vi "Send Message.vi"(6 "timeout in ms (-1)":i32=-1, 8 "error in (no error)":errorcluster, 9 "Message in":refnum<class "Abstract Message.lvclass">, 10 "Consumer in":string, 11 "Abstract Producer in":refnum<class "Abstract Producer.lvclass">) -> (0 "error out":errorcluster, 1 "Message out":refnum<class "Abstract Message.lvclass">, 3 "Abstract Producer out":refnum<class "Abstract Producer.lvclass">, 4 "timed out?":bool)   [LabVIEW 2017, in "Messaging.lvlib" / "Abstract Producer.lvclass"]
uses:
  Abstract Producer.lvclass
  Message/Abstract Message/Abstract Message.lvclass
  Abstract Producer.lvclass/Abstract Producer.ctl
  Message Queue/Abstract Message Queue/Abstract Message Queue.lvclass
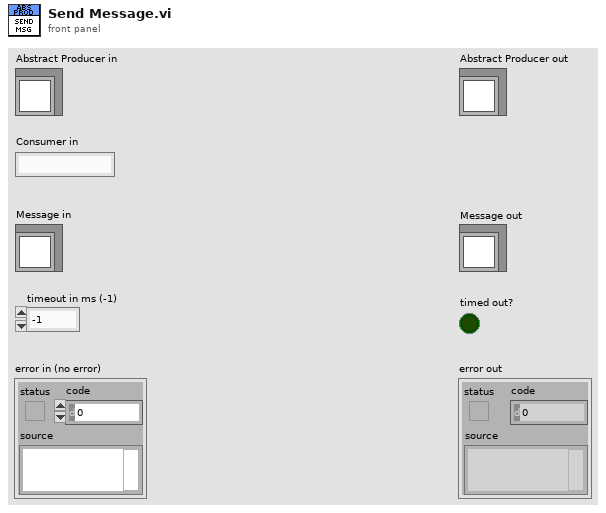
[diagram p1: front panel]
types:
  T1 = typedef "Messaging.lvlib/Abstract Producer.lvclass/Consumer Information.ctl" = cluster{"Name":string, "Request Queue":refnum<class "Abstract Message Queue.lvclass">, "Response Queue":refnum<class "Abstract Message Queue.lvclass">}
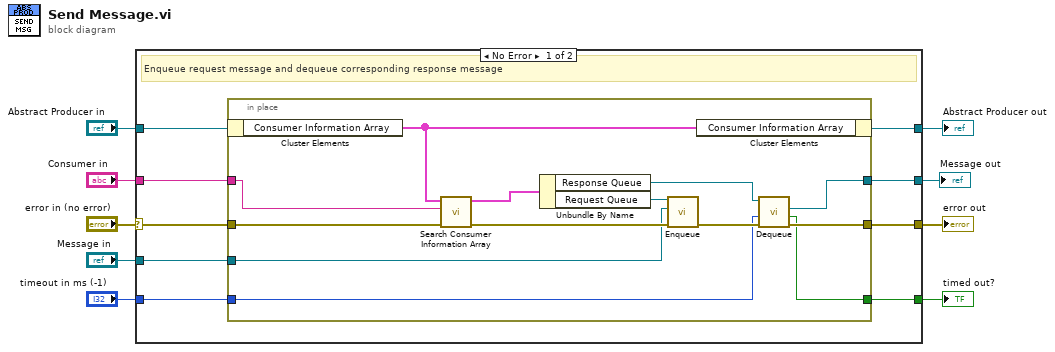
[diagram p0: block diagram]
diagram:
  n1 = case shown="No Error" "error in (no error)" {
    selector: "error in (no error)" -> [w14 w33]
    tunnel: [w13 w33] -> w8
    tunnel: [w17 w32] -> w6
    tunnel: "Abstract Producer in" -> [w18 w32]
    tunnel: "Consumer in" -> [w16 _]
    tunnel: "Message in" -> [w15 _]
    tunnel: [w12 _] -> w3
    tunnel: "timeout in ms (-1)" -> [w11 _]
    tunnel: [w10 _] -> w1
    frame No Error {
      # "Enqueue request message and dequeue corresponding response message"
      n2 = in-place {
        in-place-border: w16 -> [w31]
        in-place-border: w15 -> [w25]
        in-place-border: w14 -> [w29]
        in-place-border: [w23] -> w13
        in-place-border: [w21] -> w12
        in-place-border: w11 -> [w20]
        in-place-border: [w19] -> w10
        n3 = in-place-cluster #1(w18) -> ("Consumer Information Array"=w30:T1[])
        n4 = call "Search Consumer Information Array.vi"("error in (no error)"=w29, "Consumer in"=w31, "Consumer Information Array in"=w30) -> ("error out"=w28:errorcluster, "Consumer Information out"=w27:T1)  [unwired: 7 in]
        n5 = Unbundle By Name(w27) -> ("Response Queue"=w22:refnum<class "Abstract Message Queue.lvclass">, "Request Queue"=w26:refnum<class "Abstract Message Queue.lvclass">)
        n6 = call-dynamic "Enqueue.vi"("error in (no error)"=w28, "Message in"=w25, "Abstract Message Queue in"=w26) -> ("error out"=w24:errorcluster)  [unwired: 7 in, 1 out]
        n7 = in-place-cluster #1("Consumer Information Array"=w30) -> (w17:refnum<class "Abstract Producer.lvclass">)
        n8 = call-dynamic "Dequeue.vi"("error in (no error)"=w24, "timeout in ms (-1)"=w20, "Abstract Message Queue in"=w22) -> ("error out"=w23:errorcluster, "timed out?"=w19:bool, "Message out"=w21:refnum<class "Abstract Message.lvclass">)  [unwired: 5 in, 1 out]
      }
    }
    frame Error {
    }
  }
  "error out" <- w8
  "Abstract Producer out" <- w6
  "Message out" <- w3
  "timed out?" <- w1
